vi "ITC 503 -- upload PID table.vi"(8 "error in":errorcluster, 9 "temperature":dbl, 10 "PID table":dbl[][](array[numeric])=[[400.0, 10.0, 3.0, 1.0], [300.0, 10.0, 3.0, 1.0], [60.0, 10.0, 3.0, 1.0], [40.0, 10.0, 3.0, 1.0], [20.0, 30.0, 0.5, 0.2], [10.0, 40.0, 0.5, 0.2], [1.0, 50.0, 0.2, 0.2], [0.0, 50.0, 0.2, 0.2]], 11 "ITC503 Address":refnum<visa-resource-name>="GPIB0::24::INSTR") -> (0 "error out":errorcluster, 3 "ITC503 Address OUT":refnum<visa-resource-name>="GPIB0::24::INSTR")   [LabVIEW 2010]
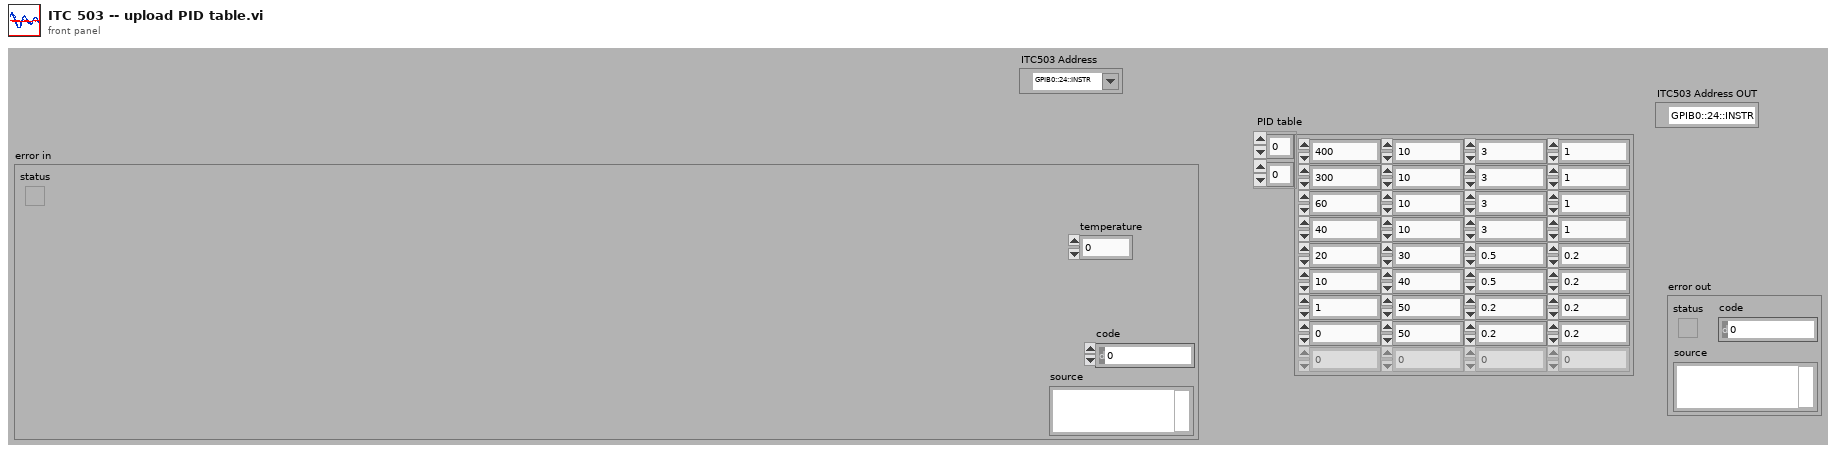
[diagram p1: front panel]
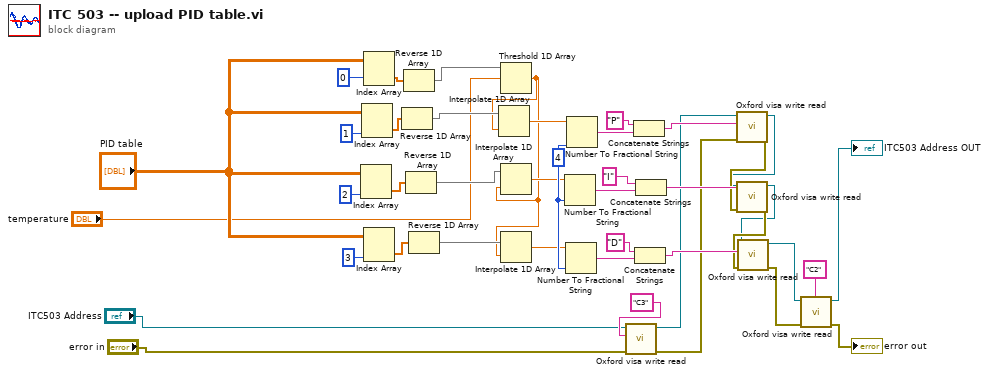
[diagram p0: block diagram]
diagram:
  w34 = i16 4 ("width (-)")
  n1 = Index Array(array="PID table", index (col)=2 ("disabled index (col)")) -> (element=w40:dbl[])  [unwired: 1 in]
  n2 = Index Array(array="PID table", index (col)=1 ("disabled index (col)")) -> (element=w41:dbl[])  [unwired: 1 in]
  n3 = Index Array(array="PID table", index (col)=0 ("disabled index (col)")) -> (element=w35:dbl[])  [unwired: 1 in]
  n4 = Index Array(array="PID table", index (col)=3 ("disabled index (col)")) -> (element=w37:dbl[])  [unwired: 1 in]
  n5 = Reverse 1D Array(array=w41) -> (reversed array=w42:dbl[])
  n6 = Reverse 1D Array(array=w35) -> (reversed array=w36:dbl[])
  n7 = Reverse 1D Array(array=w40) -> (reversed array=w39:dbl[])
  n8 = Reverse 1D Array(array=w37) -> (reversed array=w38:dbl[])
  n9 = Threshold 1D Array(2:"temperature", 3:w36) -> (0:w19:dbl)  [unwired: 1 in]
  n10 = Interpolate 1D Array(1:w19, 2:w42) -> (0:w20:dbl)
  n11 = Interpolate 1D Array(1:w19, 2:w39) -> (0:w21:dbl)
  n12 = Interpolate 1D Array(1:w19, 2:w38) -> (0:w22:dbl)
  n13 = Number To Fractional String(number=w21, precision (6)=w34) -> (F-format string=w33:string)  [unwired: 2 in]
  n14 = Number To Fractional String(number=w22, precision (6)=w34) -> (F-format string=w32:string)  [unwired: 2 in]
  n15 = Number To Fractional String(number=w20, precision (6)=w34) -> (F-format string=w23:string)  [unwired: 2 in]
  n16 = call "Oxford visa write read.vi"("error in (no error)"="error in", "write buffer"="C3" ("Command"), "VISA resource name"="ITC503 Address") -> ("error out"=w14:errorcluster, "VISA resource name out"=w6:refnum<visa-resource-name>)  [unwired: 6 in, 1 out]
  n17 = Concatenate Strings("P" ("string"), w23) -> (w29:string)
  n18 = Concatenate Strings("D" ("string"), w32) -> (w31:string)
  n19 = Concatenate Strings("I" ("string"), w33) -> (w30:string)
  n20 = call "Oxford visa write read.vi"("error in (no error)"=w14, "write buffer"=w29, "VISA resource name"=w6) -> ("error out"=w27:errorcluster, "VISA resource name out"=w5:refnum<visa-resource-name>)  [unwired: 6 in, 1 out]
  n21 = call "Oxford visa write read.vi"("error in (no error)"=w27, "write buffer"=w30, "VISA resource name"=w5) -> ("error out"=w28:errorcluster, "VISA resource name out"=w4:refnum<visa-resource-name>)  [unwired: 6 in, 1 out]
  n22 = call "Oxford visa write read.vi"("error in (no error)"=w28, "write buffer"=w31, "VISA resource name"=w4) -> ("error out"=w11:errorcluster, "VISA resource name out"=w3:refnum<visa-resource-name>)  [unwired: 6 in, 1 out]
  n23 = call "Oxford visa write read.vi"("error in (no error)"=w11, "write buffer"="C2" ("Command"), "VISA resource name"=w3) -> ("error out"=→"error out":errorcluster, "VISA resource name out"=→"ITC503 Address OUT":refnum<visa-resource-name>)  [unwired: 6 in, 1 out]
